vi "SendDatabase2Cerebus.vi"(1 "Database":T1={"ExperimentDate"=timestamp(3401900640.652657 s since 1904-01-01), "ImplantDate"=timestamp(3401876933.0000005 s since 1904-01-01), "CerebusFolder"="", "Experimenter"="Tyler Davis", "PatientNumber"="201102", "DominantHand"="Right", "DeviceType"="uECOG", "DeviceSerial"="CG-64BPX-F419", "DeviceHemisphere"="Right", "DeviceRegion"="Motor", "TaskType"="FingerPressTask.vi", "TaskComments"="", "RecordingComments"="", "GeneralObservations"=""}) -> (0 "ParameterString":string)   [LabVIEW 2011]
panel:
  # "Do not place ';' or '=' in the comment fields"
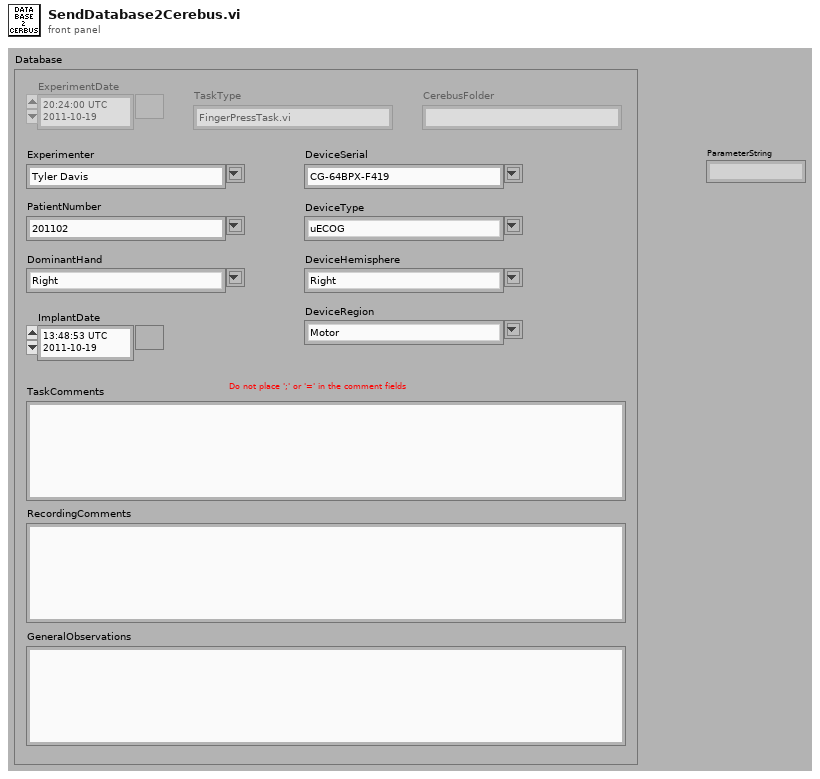
[diagram p1: front panel]
types:
  T1 = cluster{"ExperimentDate":timestamp, "ImplantDate":timestamp, "CerebusFolder":string, "Experimenter":string, "PatientNumber":string, "DominantHand":string, "DeviceType":string, "DeviceSerial":string, "DeviceHemisphere":string, "DeviceRegion":string, "TaskType":string, "TaskComments":string, "RecordingComments":string, "GeneralObservations":string}
  T2 = enum16{"Initialize", "String", "Start", "New Session", "Stop", "Resume", "Close"}
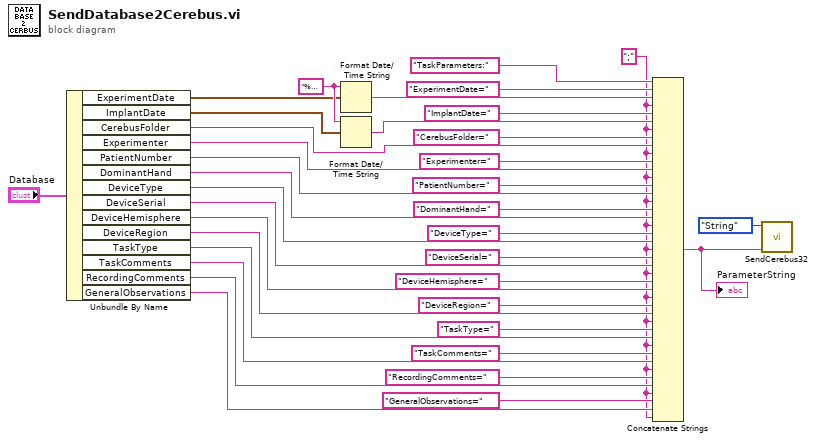
[diagram p0: block diagram]
diagram:
  w4 = ";" ("element")
  w10 = "%Y%m%d-%H%M%S" ("time format string (%c)")
  n1 = Unbundle By Name("Database") -> ("ExperimentDate"=w8:timestamp, "ImplantDate"=w9:timestamp, "CerebusFolder"=w26:string, "Experimenter"=w27:string, "PatientNumber"=w28:string, "DominantHand"=w29:string, "DeviceType"=w30:string, "DeviceSerial"=w31:string, "DeviceHemisphere"=w32:string, "DeviceRegion"=w33:string, "TaskType"=w34:string, "TaskComments"=w35:string, "RecordingComments"=w36:string, "GeneralObservations"=w5:string)
  n2 = Format Date/Time String(time format string (%c)=w10, seconds (now)=w8) -> (date/time string=w24:string)  [unwired: 1 in]
  n3 = Format Date/Time String(time format string (%c)=w10, seconds (now)=w9) -> (date/time string=w25:string)  [unwired: 1 in]
  n4 = Concatenate Strings("TaskParameters:" ("string"), "ExperimentDate=" ("string"), w24, w4, "ImplantDate=" ("string"), w25, w4, "CerebusFolder=" ("string"), w26, w4, "Experimenter=" ("string"), w27, w4, "PatientNumber=" ("string"), w28, w4, "DominantHand=" ("string"), w29, w4, "DeviceType=" ("string"), w30, w4, "DeviceSerial=" ("string"), w31, w4, "DeviceHemisphere=" ("string"), w32, w4, "DeviceRegion=" ("string"), w33, w4, "TaskType=" ("string"), w34, w4, "TaskComments=" ("string"), w35, w4, "RecordingComments=" ("string"), w36, w4, "GeneralObservations=" ("string"), w5, w4) -> (w2:string)
  "ParameterString" <- w2
  n5 = call "SendCerebus32.vi"("String"=w2, "Mode"=T2."String") -> ()  [unwired: 3 in]
